vi "_TangoDeviceAttributesList.vi"(2 "error in":errorcluster, 3 "device name":string) -> (0 "error out":errorcluster, 1 "attributes_list":string[](array[string]))   [LabVIEW 2014, in "tango.lvlib"]
uses:
  tango.lvlib
  tango_binding.so
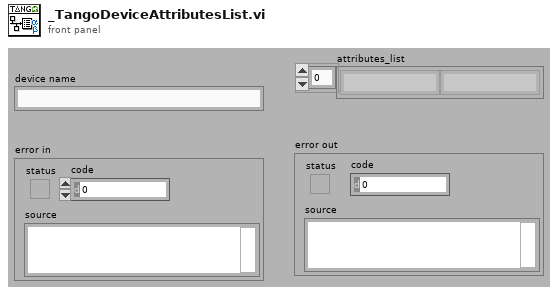
[diagram p1: front panel]
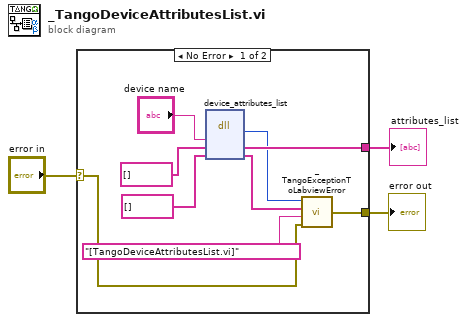
[diagram p0: block diagram]
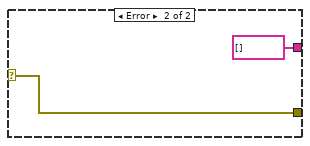
[diagram p2: hidden frame]
diagram:
  n1 = case shown="No Error" "error in" {
    selector: "error in" -> [w4 w14]
    tunnel: [w12 string[] [] ("attributes_list")] -> w3
    tunnel: [w8 w14] -> w2
    frame No Error {
      n2 = dll-call lib="tango_binding.*" fn="device_attributes_list"("dev_name"="device name", "attributes_list"=string[] [] ("Error Stack"), "error_stack"=string[] [] ("Error Stack")) -> ("return type"=w6:i32, "attributes_list"=w12:string[], "error_stack"=w7:string[])  [unwired: 4 in, 2 out]
      n3 = call "_TangoExceptionToLabviewError.vi"("error in"=w4, "location"="[TangoDeviceAttributesList.vi]", "error stack"=w7, "error code"=w6) -> ("error out"=w8:errorcluster)
    }
    frame Error {
    }
  }
  "attributes_list" <- w3
  "error out" <- w2
